vi "duration text to number.vi"(1 "durations (ms)":string[](array[string])) -> (0 "durations2 (ms)":dbl[](array[numeric]) format="%.2f")   [LabVIEW 2017]
doc: "This vi identifies variables appear in durations, and convert the string format durations to real number durations"
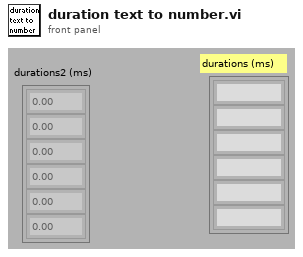
[diagram p1: front panel]
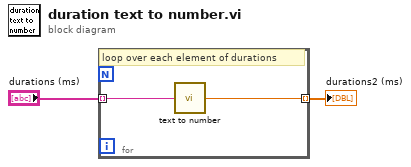
[diagram p0: block diagram]
diagram:
  n1 = for {
    tunnel: "durations (ms)" -> [w4] mode=indexing
    tunnel: [w3] -> w1 mode=indexing
    # "loop over each element of durations"
    n2 = call "text to number.vi"("text"=w4) -> ("number"=w3:dbl)
  }
  "durations2 (ms)" <- w1
